vi "Tool offset Calculator.vi"() -> ()   [LabVIEW 2011]
uses:
  Shared Components/Gantry Class/Type Definitions/Virtual Modes.ctl
  Shared Components/Gantry Class/Type Definitions/Init_Modes.ctl
  Shared Components/Config Manager Class/Type Definitions/Camera Enum.ctl
  Shared Components/Gantry Class/Gantry Class.lvclass
  Shared Components/Vec3d Class/Vec3d Class.lvclass
panel:
  in  "Virtual Mode":T1=enum."Virtual"
  in  "stop":bool
  out "Image":T2(plugin-control)
  out "error out":errorcluster
  in  "Config Folder":path=path "C:/Users/Admin/Gantry Purdue/pixel-gantry-control/Config"
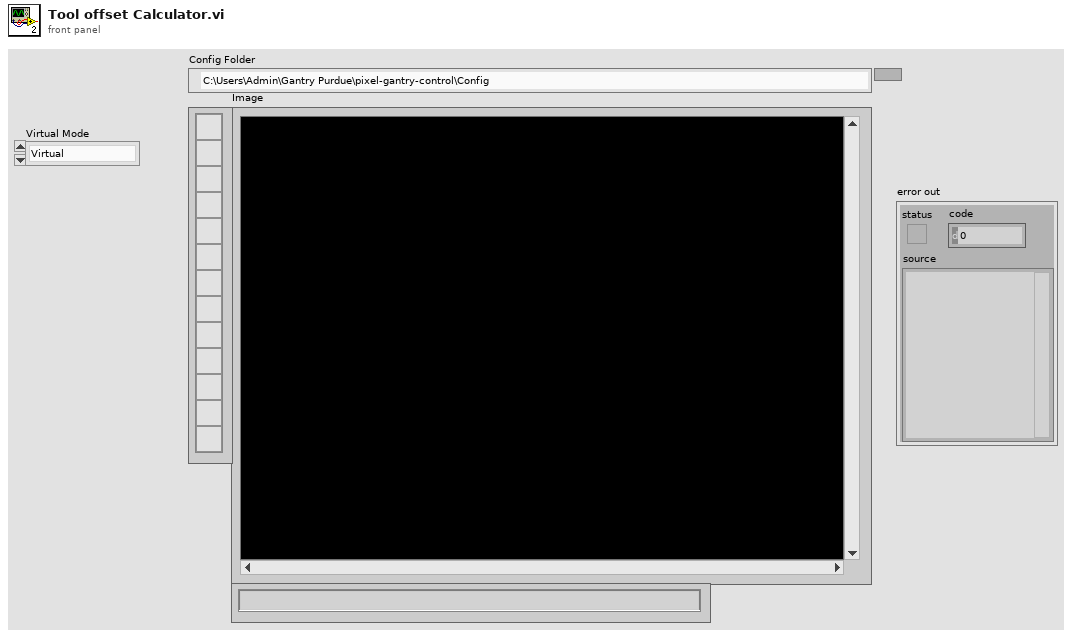
[diagram p1: front panel]
types:
  T1 = typedef "Virtual Modes.ctl" = enum16{"Nonvirtual", "Pseudovirtual", "Virtual"}
  T2 = typedef "IMAQ Image.ctl" = refnum<image>
  T3 = typedef "Camera Enum.ctl" = enum16{"GANTRY HEAD", "NEEDLE CALIBRATION X", "NEEDLE CALIBRATION Y", "STAND CAMERA", "SIMRAN WEBCAM"}
  T4 = typedef "Init_Modes.ctl" = enum16{"Full", "Robot Only", "Dispenser Only", "Cameras Only", "Robot and Cameras", "Robot and Cameras and Dispenser", "Manifold Only"}
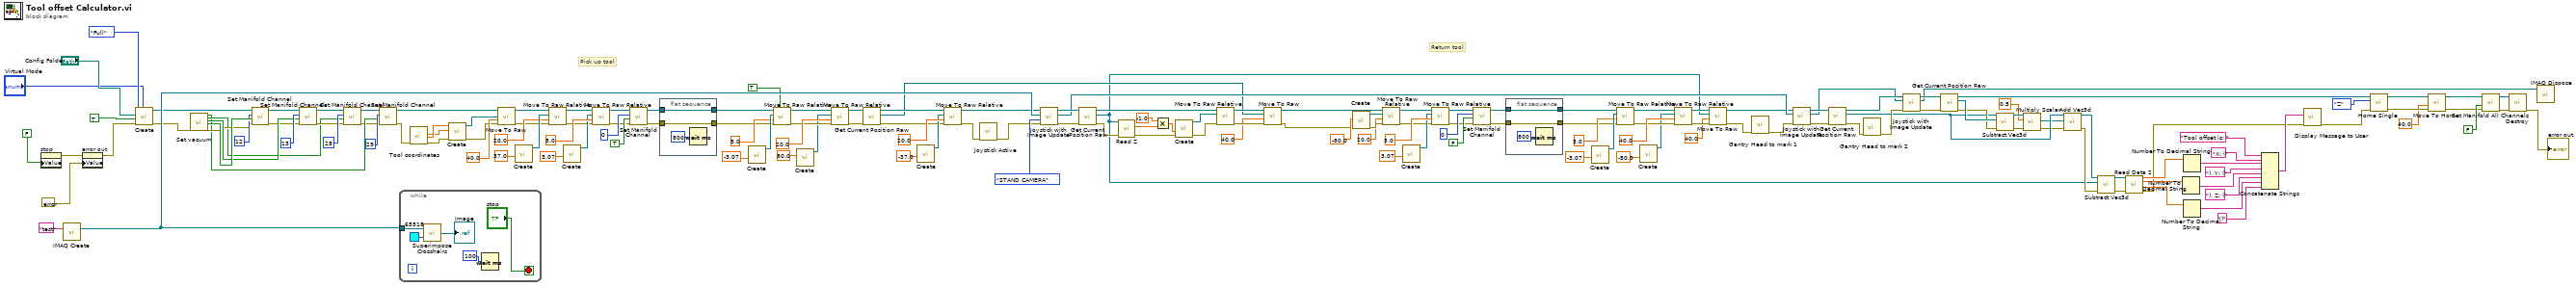
[diagram p0: block diagram]
diagram:
  # "Return tool"
  # "Pick up tool"
  n1 = property on="stop" class="Bool (strict)"("Value"=FALSE) -> (error out=w160:errorcluster)  [unwired: 2 in, 1 out]
  n2 = call "IMAQ Create"("Image Name"="test") -> ("New Image"=w163:T2)  [unwired: 4 in, 1 out]
  n3 = property on="error out" class="Clust (strict)"(error in=w160, "Value"=errorcluster {"status"=FALSE, "code"=0, "source"=""} ("error in (no error)")) -> (error out=w159:errorcluster)  [unwired: 1 in, 1 out]
  n4 = call "Create.vi"("Virtual Mode"="Virtual Mode", "error in"=w159, "HOME?"=TRUE, "Config Folder"="Config Folder", "Init Mode"=Init_Modes."Full") -> ("error out"=w7:errorcluster, "Gantry out"=w9:refnum<class "Gantry Class.lvclass">)  [unwired: 5 in]
  n5 = call "Set vacuum"("error in (no error)"=w7) -> ("Vacuum 2B"=w11:bool, "Vacuum 2A"=w13:bool, "Vacuum 1B"=w18:bool, "Vacuum 1A"=w24:bool, "error out"=w17:errorcluster)  [unwired: 13 in, 1 out]
  n6 = call-dynamic "Set Manifold Channel.vi"("error in"=w17, "On/Off"=w24, "Manifold Channel"=12, "Gantry in"=w9) -> ("error out"=w16:errorcluster, "Gantry out"=w19:refnum<class "Gantry Class.lvclass">)  [unwired: 6 in]
  n7 = call-dynamic "Set Manifold Channel.vi"("error in"=w16, "On/Off"=w18, "Manifold Channel"=13, "Gantry in"=w19) -> ("error out"=w15:errorcluster, "Gantry out"=w14:refnum<class "Gantry Class.lvclass">)  [unwired: 6 in]
  n8 = call-dynamic "Set Manifold Channel.vi"("error in"=w15, "On/Off"=w13, "Manifold Channel"=28, "Gantry in"=w14) -> ("error out"=w10:errorcluster, "Gantry out"=w12:refnum<class "Gantry Class.lvclass">)  [unwired: 6 in]
  n9 = call-dynamic "Set Manifold Channel.vi"("error in"=w10, "On/Off"=w11, "Manifold Channel"=29, "Gantry in"=w12) -> ("error out"=w6:errorcluster, "Gantry out"=w8:refnum<class "Gantry Class.lvclass">)  [unwired: 6 in]
  n10 = while {
    tunnel: w163 -> [w170]
    stop <- "stop" stop-if-true
    n11 = call "Superimpose Crosshairs.vi"("Grid Line Color"=u32 65518, "Refnum in"=w170) -> ("Refnum out"=→"Image":T2)
    n12 = Wait (ms)(milliseconds to wait=u32 100) -> ()  [unwired: 1 out]
  }
  n13 = call "Tool coordinates"("error in (no error)"=w6) -> ("Y"=w154:dbl, "X"=w155:dbl, "error out"=w151:errorcluster)  [unwired: 15 in, 1 out]
  n14 = call "Create.vi"("error in"=w151, "Y"=w154, "X"=w155) -> ("error out"=w152:errorcluster, "Vec3d Class out"=w84:refnum<class "Vec3d Class.lvclass">)  [unwired: 7 in]
  n15 = call-dynamic "Move To Raw.vi"("error in"=w152, "Speed"=40.0, "Destination"=w84, "Gantry in"=w8) -> ("error out"=w134:errorcluster, "Gantry out"=w143:refnum<class "Gantry Class.lvclass">)  [unwired: 6 in]
  n16 = call "Create.vi"("Z"=37.0) -> ("Vec3d Class out"=w145:refnum<class "Vec3d Class.lvclass">)  [unwired: 9 in, 1 out]
  n17 = call-dynamic "Move To Raw Relative.vi"("Speed(mm/s)"=20.0, "Delta"=w145, "Gantry in"=w143) -> ("Gantry out"=w136:refnum<class "Gantry Class.lvclass">)  [unwired: 7 in, 1 out]
  n18 = call "Create.vi"("Z"=3.07) -> ("Vec3d Class out"=w137:refnum<class "Vec3d Class.lvclass">)  [unwired: 9 in, 1 out]
  n19 = call-dynamic "Move To Raw Relative.vi"("error in"=w134, "Speed(mm/s)"=5.0, "Delta"=w137, "Gantry in"=w136) -> ("error out"=w133:errorcluster, "Gantry out"=w135:refnum<class "Gantry Class.lvclass">)  [unwired: 6 in]
  n20 = call-dynamic "Set Manifold Channel.vi"("error in"=w133, "On/Off"=TRUE, "Manifold Channel"=0, "Gantry in"=w135) -> ("error out"=w38:errorcluster, "Gantry out"=w40:refnum<class "Gantry Class.lvclass">)  [unwired: 6 in]
  n21 = flat-sequence {
    tunnel: w40 -> [w175]
    tunnel: [w175] -> w39
    tunnel: w38 -> [w173]
    tunnel: [w173] -> w37
    frame #0 {
      n22 = Wait (ms)(milliseconds to wait=u32 800) -> ()  [unwired: 1 out]
    }
  }
  n23 = call "Create.vi"("Z"=-3.07) -> ("Vec3d Class out"=w131:refnum<class "Vec3d Class.lvclass">)  [unwired: 9 in, 1 out]
  n24 = call-dynamic "Move To Raw Relative.vi"("Wait?"=TRUE, "error in"=w37, "Speed(mm/s)"=5.0, "Delta"=w131, "Gantry in"=w39) -> ("error out"=w126:errorcluster, "Gantry out"=w127:refnum<class "Gantry Class.lvclass">)  [unwired: 5 in]
  n25 = call "Create.vi"("Y"=80.0 ("Z")) -> ("Vec3d Class out"=w125:refnum<class "Vec3d Class.lvclass">)  [unwired: 9 in, 1 out]
  n26 = call-dynamic "Move To Raw Relative.vi"("error in"=w126, "Speed(mm/s)"=20.0, "Delta"=w125, "Gantry in"=w127) -> ("error out"=w71:errorcluster, "Gantry out"=w73:refnum<class "Gantry Class.lvclass">)  [unwired: 6 in]
  n27 = call-dynamic "Get Current Position Raw.vi"("error in"=w71, "Gantry in"=w73) -> ("error out"=w70:errorcluster, "Vec3d Class out"=w68:refnum<class "Vec3d Class.lvclass">, "Gantry out"=w72:refnum<class "Gantry Class.lvclass">)  [unwired: 7 in]
  n28 = call "Create.vi"("Z"=-37.0) -> ("Vec3d Class out"=w121:refnum<class "Vec3d Class.lvclass">)  [unwired: 9 in, 1 out]
  n29 = call-dynamic "Move To Raw Relative.vi"("error in"=w70, "Speed(mm/s)"=20.0, "Delta"=w121, "Gantry in"=w72) -> ("error out"=w119:errorcluster, "Gantry out"=w120:refnum<class "Gantry Class.lvclass">)  [unwired: 6 in]
  n30 = call "Joystick Active"("error in (no error)"=w119) -> ("error out"=w118:errorcluster)  [unwired: 17 in, 1 out]
  n31 = call-dynamic "Joystick with Image Update.vi"("error in (no error)"=w118, "Camera Name"=Camera_Enum."STAND CAMERA", "Image In"=w163, "Gantry Class in"=w120) -> ("error out"=w148:errorcluster, "Image Out"=w117:T2, "Gantry Class out"=w149:refnum<class "Gantry Class.lvclass">)  [unwired: 5 in]
  n32 = call-dynamic "Get Current Position Raw.vi"("error in"=w148, "Gantry in"=w149) -> ("error out"=w83:errorcluster, "Vec3d Class out"=w42:refnum<class "Vec3d Class.lvclass">, "Gantry out"=w80:refnum<class "Gantry Class.lvclass">)  [unwired: 7 in]
  n33 = call-dynamic "Read Z.vi"("error in (no error)"=w83, "Vec3d Class in"=w42) -> ("error out"=w79:errorcluster, "Z"=w82:dbl)  [unwired: 7 in, 1 out]
  n34 = Multiply(x=-1.0, y=w82) -> (x*y=w78:dbl)
  n35 = call "Create.vi"("error in"=w79, "Z"=w78) -> ("error out"=w76:errorcluster, "Vec3d Class out"=w77:refnum<class "Vec3d Class.lvclass">)  [unwired: 8 in]
  n36 = call-dynamic "Move To Raw Relative.vi"("error in"=w76, "Delta"=w77, "Gantry in"=w80) -> ("error out"=w75:errorcluster, "Gantry out"=w74:refnum<class "Gantry Class.lvclass">)  [unwired: 7 in]
  n37 = call-dynamic "Move To Raw.vi"("error in"=w75, "Speed"=40.0, "Destination"=w68, "Gantry in"=w74) -> ("error out"=w32:errorcluster, "Gantry out"=w31:refnum<class "Gantry Class.lvclass">)  [unwired: 6 in]
  n38 = call "Create.vi"("error in"=w32, "Y"=-80.0) -> ("error out"=w67:errorcluster, "Vec3d Class out"=w41:refnum<class "Vec3d Class.lvclass">)  [unwired: 8 in]
  n39 = call-dynamic "Move To Raw Relative.vi"("error in"=w67, "Speed(mm/s)"=20.0, "Delta"=w41, "Gantry in"=w31) -> ("error out"=w49:errorcluster, "Gantry out"=w50:refnum<class "Gantry Class.lvclass">)  [unwired: 6 in]
  n40 = call "Create.vi"("Z"=3.07) -> ("Vec3d Class out"=w60:refnum<class "Vec3d Class.lvclass">)  [unwired: 9 in, 1 out]
  n41 = call-dynamic "Move To Raw Relative.vi"("error in"=w49, "Speed(mm/s)"=5.0, "Delta"=w60, "Gantry in"=w50) -> ("error out"=w58:errorcluster, "Gantry out"=w59:refnum<class "Gantry Class.lvclass">)  [unwired: 6 in]
  n42 = call-dynamic "Set Manifold Channel.vi"("error in"=w58, "On/Off"=FALSE, "Manifold Channel"=0, "Gantry in"=w59) -> ("error out"=w34:errorcluster, "Gantry out"=w36:refnum<class "Gantry Class.lvclass">)  [unwired: 6 in]
  n43 = flat-sequence {
    tunnel: w36 -> [w178]
    tunnel: [w178] -> w35
    tunnel: w34 -> [w176]
    tunnel: [w176] -> w33
    frame #0 {
      n44 = Wait (ms)(milliseconds to wait=u32 800) -> ()  [unwired: 1 out]
    }
  }
  n45 = call "Create.vi"("Z"=-3.07) -> ("Vec3d Class out"=w56:refnum<class "Vec3d Class.lvclass">)  [unwired: 9 in, 1 out]
  n46 = call-dynamic "Move To Raw Relative.vi"("error in"=w33, "Speed(mm/s)"=5.0, "Delta"=w56, "Gantry in"=w35) -> ("error out"=w52:errorcluster, "Gantry out"=w53:refnum<class "Gantry Class.lvclass">)  [unwired: 6 in]
  n47 = call "Create.vi"("Z"=-50.0) -> ("Vec3d Class out"=w51:refnum<class "Vec3d Class.lvclass">)  [unwired: 9 in, 1 out]
  n48 = call-dynamic "Move To Raw Relative.vi"("error in"=w52, "Speed(mm/s)"=40.0, "Delta"=w51, "Gantry in"=w53) -> ("error out"=w46:errorcluster, "Gantry out"=w47:refnum<class "Gantry Class.lvclass">)  [unwired: 6 in]
  n49 = call-dynamic "Move To Raw.vi"("error in"=w46, "Speed"=40.0, "Destination"=w42, "Gantry in"=w47) -> ("error out"=w43:errorcluster, "Gantry out"=w44:refnum<class "Gantry Class.lvclass">)  [unwired: 6 in]
  n50 = call "Gantry Head to mark 1"("error in (no error)"=w43) -> ("error out"=w156:errorcluster)  [unwired: 9 in, 1 out]
  n51 = call-dynamic "Joystick with Image Update.vi"("error in (no error)"=w156, "Image In"=w117, "Gantry Class in"=w44) -> ("error out"=w161:errorcluster, "Image Out"=w93:T2, "Gantry Class out"=w162:refnum<class "Gantry Class.lvclass">)  [unwired: 6 in]
  n52 = call-dynamic "Get Current Position Raw.vi"("error in"=w161, "Gantry in"=w162) -> ("error out"=w112:errorcluster, "Vec3d Class out"=w106:refnum<class "Vec3d Class.lvclass">, "Gantry out"=w113:refnum<class "Gantry Class.lvclass">)  [unwired: 7 in]
  n53 = call "Gantry Head to mark 2"("error in (no error)"=w112) -> ("error out"=w114:errorcluster)  [unwired: 9 in, 1 out]
  n54 = call-dynamic "Joystick with Image Update.vi"("error in (no error)"=w114, "Image In"=w93, "Gantry Class in"=w113) -> ("error out"=w115:errorcluster, "Image Out"=w92:T2, "Gantry Class out"=w116:refnum<class "Gantry Class.lvclass">)  [unwired: 6 in]
  n55 = call-dynamic "Get Current Position Raw.vi"("error in"=w115, "Gantry in"=w116) -> ("error out"=w110:errorcluster, "Vec3d Class out"=w111:refnum<class "Vec3d Class.lvclass">, "Gantry out"=w29:refnum<class "Gantry Class.lvclass">)  [unwired: 7 in]
  n56 = call "Subtract Vec3d.vi"("error in (no error)"=w110, "Vec3d in 2"=w111, "Vec3d in 1"=w106) -> ("error out"=w108:errorcluster, "Vec3d Class out"=w109:refnum<class "Vec3d Class.lvclass">)  [unwired: 7 in]
  n57 = call-dynamic "Multiply Scalar.vi"("error in"=w108, "Scale"=0.5, "Vec3d in"=w109) -> ("error out"=w104:errorcluster, "Vec3d out"=w105:refnum<class "Vec3d Class.lvclass">)  [unwired: 7 in]
  n58 = call-dynamic "Add Vec3d.vi"("error in (no error)"=w104, 10:"Vec3d Class in"=w105, 11:"Vec3d Class in"=w106) -> ("error out"=w102:errorcluster, "Vec3d Class out"=w103:refnum<class "Vec3d Class.lvclass">)  [unwired: 7 in]
  n59 = call "Subtract Vec3d.vi"("error in (no error)"=w102, "Vec3d in 2"=w42, "Vec3d in 1"=w103) -> ("error out"=w100:errorcluster, "Vec3d Class out"=w101:refnum<class "Vec3d Class.lvclass">)  [unwired: 7 in]
  n60 = call-dynamic "Read Data 2.vi"("error in"=w100, "Vec3d in"=w101) -> ("error out"=w94:errorcluster, "Z"=w97:dbl, "Y"=w98:dbl, "X"=w99:dbl)  [unwired: 6 in]
  n61 = Number To Decimal String(number=w98) -> (decimal integer string=w91:string)  [unwired: 1 in]
  n62 = Number To Decimal String(number=w99) -> (decimal integer string=w96:string)  [unwired: 1 in]
  n63 = Number To Decimal String(number=w97) -> (decimal integer string=w87:string)  [unwired: 1 in]
  n64 = Concatenate Strings("Tool offset is: " ("string"), "X: (" ("string"), w96, "), Y: (" ("string"), w91, "), Z: (" ("string"), w87, ")" ("string")) -> (w95:string)
  n65 = call "Display Message to User"("error in (no error)"=w94, "Message"=w95) -> ("error out"=w28:errorcluster)  [unwired: 8 in, 1 out]
  n66 = call-dynamic "Home Single.vi"("error in"=w28, "Axis"=enum16{"X", "Y", "Z", "U"}."Z", "Gantry in"=w29) -> ("error out"=w26:errorcluster, "Gantry out"=w27:refnum<class "Gantry Class.lvclass">)  [unwired: 7 in]
  n67 = call-dynamic "Move To Home.vi"("error in"=w26, "Speed(mm/s)"=40.0, "Gantry in"=w27) -> ("error out"=w3:errorcluster, "Gantry out"=w4:refnum<class "Gantry Class.lvclass">)  [unwired: 7 in]
  n68 = call-dynamic "Set Manifold All Channels.vi"("error in"=w3, "On/Off"=FALSE, "Gantry in"=w4) -> ("error out"=w2:errorcluster, "Gantry out"=w1:refnum<class "Gantry Class.lvclass">)  [unwired: 7 in]
  n69 = call "Destroy.vi"("error in"=w2, "Gantry Class in"=w1) -> ("error out"=→"error out":errorcluster)  [unwired: 9 in]
  n70 = call "IMAQ Dispose"("Image"=w92) -> ()  [unwired: 5 in, 1 out]
